vi "MovePicture.vi"() -> ()   [LabVIEW 2011]
panel:
  out "new picture":picture
  in  "stop":bool
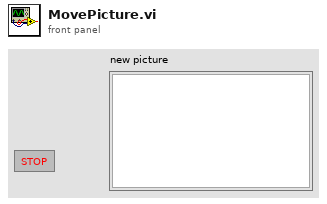
[diagram p1: front panel]
types:
  T1 = typedef "imagedata.ctl" = cluster{"image type":i32, "image depth":i32, "image":u8[], "mask":u8[], "colors":u32[], "Rectangle":cluster{"left":i16, "top":i16, "right":i16, "bottom":i16}}
  T2 = typedef "LVPoint32TypeDef.ctl" = cluster{"Horizontal":i32, "Vertical":i32}
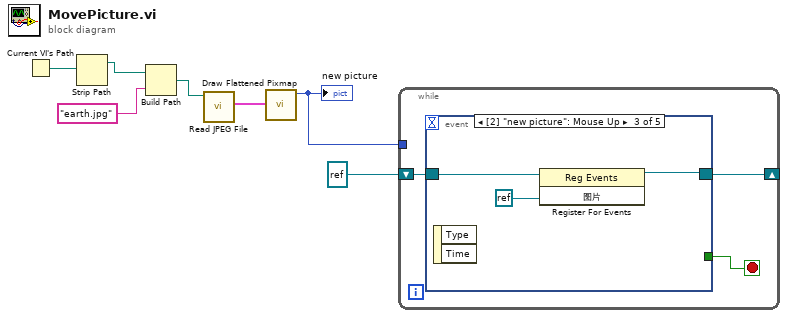
[diagram p0: block diagram]
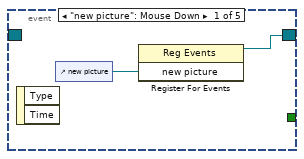
[diagram p2: hidden frame]
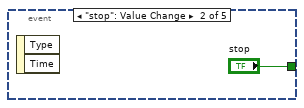
[diagram p3: hidden frame]
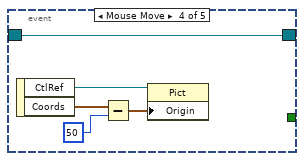
[diagram p4: hidden frame]
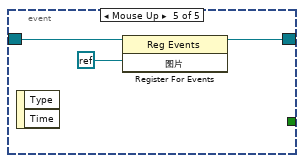
[diagram p5: hidden frame]
diagram:
  n1 = Current VI's Path() -> (path=w7:path)
  n2 = Strip Path(path=w7) -> (stripped path=w6:path)  [unwired: 1 out]
  n3 = Build Path(base path=w6, name or relative path="earth.jpg") -> (appended path=w4:path)
  n4 = call <vilib>:"Read JPEG File.vi"("path to JPEG file"=w4) -> ("image data"=w3:T1)  [unwired: 8 in, 2 out]
  n5 = call <vilib>:"Draw Flattened Pixmap.vi"("image data"=w3) -> ("new picture"=w2:picture)  [unwired: 8 in]
  "new picture" <- w2
  n6 = while {
    tunnel: w2 -> [_]
    shift-right: [w8] -> _
    shift-left: refnum<event-registration> refnum ("事件注册引用句柄") -> [w9]
    stop <- w10 stop-if-true
    n7 = event shown="[2] \"new picture\": Mouse Up" {
      selector: w9 -> [_ _ w16 w17 w24]
      dyn-events: [w11 _ w15 w17 w23] -> w8
      timeout: _ -> [_ _ _ _ _]
      tunnel: [_ "stop" _ _ _] -> w10
      event "new picture": Mouse Down {
        n8 = event-data() -> ()  [unwired: 1 in, 2 out]
        n9 = control-ref of="new picture"() -> (w12:refnum<vi>)
        n10 = register-events(w12) -> (reference out=w11:refnum<event-registration>)  [unwired: 2 in, 1 out]
      }
      event "stop": Value Change {
        n11 = event-data() -> ()  [unwired: 1 in, 2 out]
      }
      event "new picture": Mouse Up {
        n12 = event-data() -> ()  [unwired: 1 in, 2 out]
        n13 = register-events(reference=w16, refnum<k0> refnum) -> (reference out=w15:refnum<event-registration>)  [unwired: 1 in, 1 out]
      }
      event Mouse Move {
        n14 = event-data() -> ("CtlRef"=w21:refnum<vi>, "Coords"=w20:T2)  [unwired: 1 in]
        n15 = Subtract(x=w20, y=50) -> (x-y=w19:T2)
        n16 = property class="Pict"(reference=w21, "Origin"=w19) -> ()  [unwired: 1 in, 2 out]
      }
      event Mouse Up {
        n17 = event-data() -> ()  [unwired: 1 in, 2 out]
        n18 = register-events(reference=w24, refnum<k0> refnum) -> (reference out=w23:refnum<event-registration>)  [unwired: 1 in, 1 out]
      }
    }
  }
